vi "Measurement_UI.vi"() -> ()   [LabVIEW 2023]
uses:
  <vilib>/Instr/_visa.llb/VISA Configure Serial Port (Instr).vi
panel:
  in  "Automation Irrigation Systems":enum32{"Introverts' Garden"}(tab)
  out "Water Tension":dbl(graph)
  out "Water Tension (cbar)":dbl(knob) scale=10.0..200.0
  out "Temperature (C)":dbl(knob) scale=10.0..40.0
  out "Humidity (%)":dbl(knob) scale=0.0..100.0
  in  "Device PORT":refnum<visa-resource-name>
  in  "?":bool
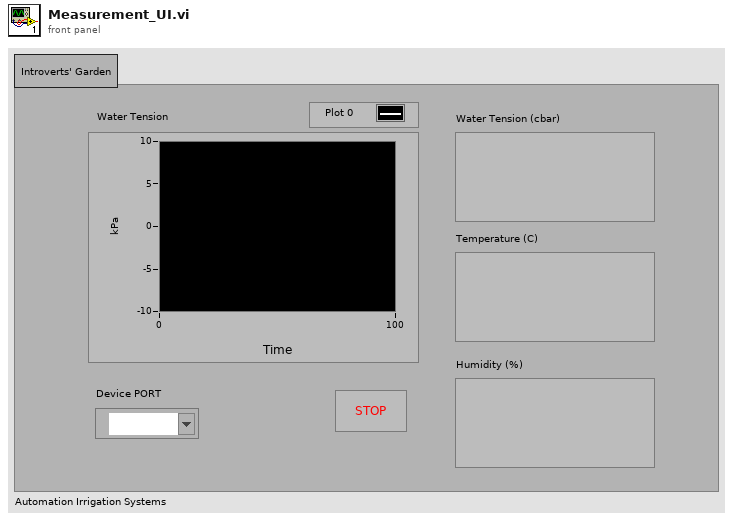
[diagram p1: front panel]
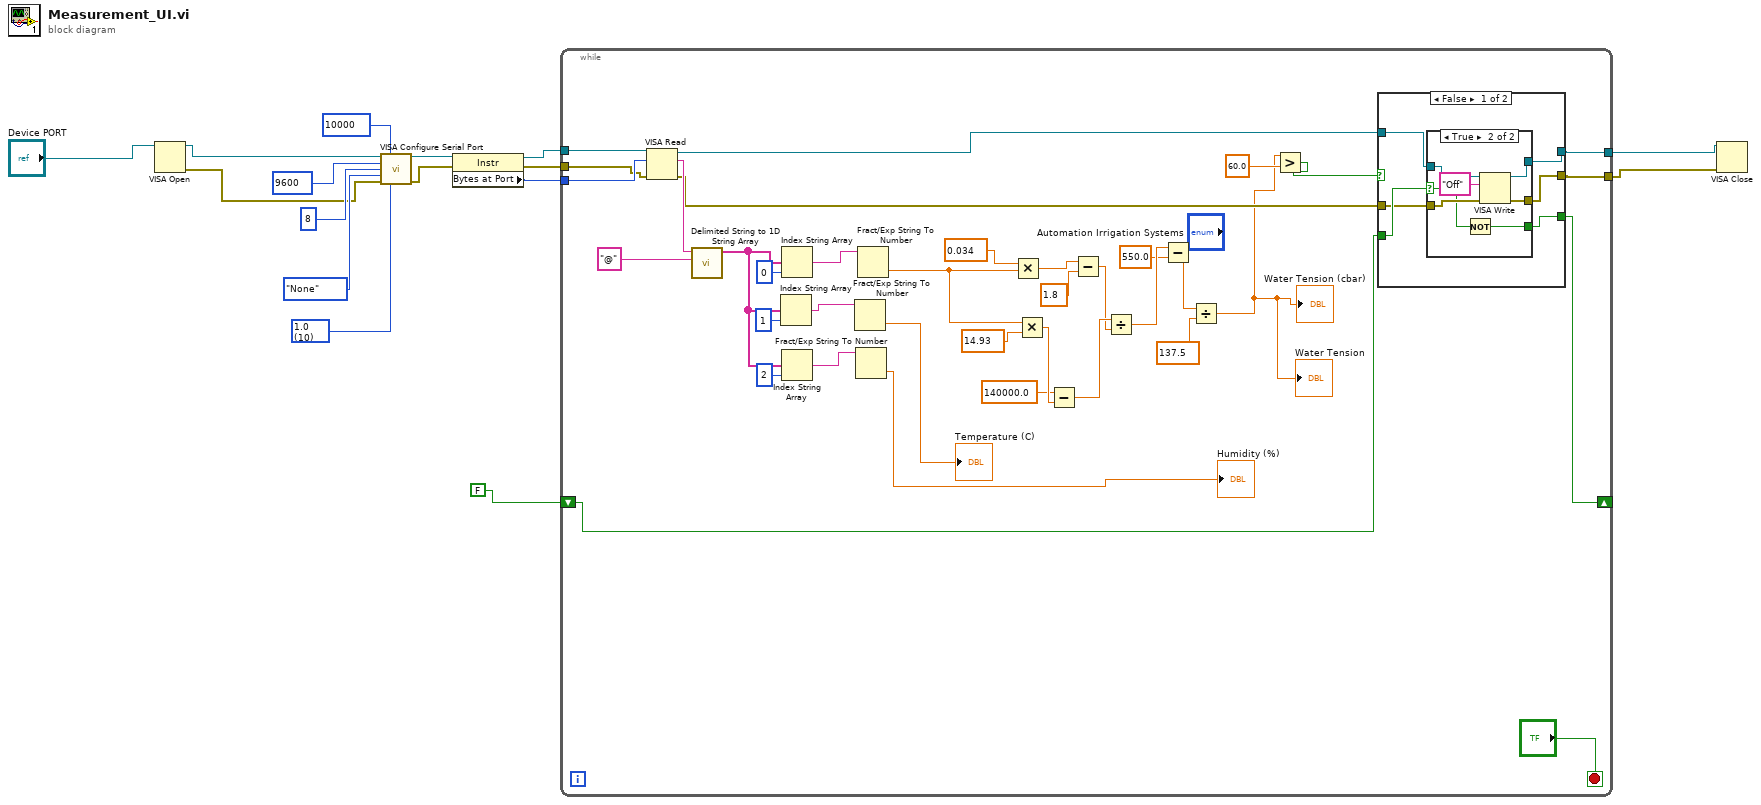
[diagram p0: block diagram]
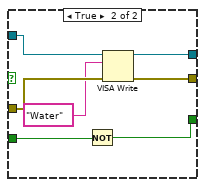
[diagram p3: hidden frame]
diagram:
  w13 = u16 10 items=["1.0"=10, "1.5"=15, "2.0"=20] ("stop bits (10: 1 bit)")
  n1 = VISA Open(VISA resource name="Device PORT") -> (VISA resource name=w10:refnum<visa-resource-name>, error out=w9:errorcluster)  [unwired: 4 in]
  n2 = call-poly "VISA Configure Serial Port"("VISA resource name"=w10, "timeout (10sec)"=u32 10000, "baud rate (9600)"=u32 9600, "data bits (8)"=u16 8, "parity (0:none)"=enum16{"None", "Odd", "Even", "Mark", "Space"}."None", "error in (no error)"=w9, "stop bits (10: 1 bit)"=w13) -> ("VISA resource name out"=w8:refnum<visa-resource-name>, "error out"=w7:errorcluster)  [unwired: 7 in]
  n3 = property class="Instr"(reference=w8, error in=w7) -> (reference out=w6:refnum<visa-resource-name>, error out=w5:errorcluster, "Bytes at Port"=w4:u32)
  n4 = while {
    tunnel: w6 -> [w53]
    tunnel: w5 -> [w51]
    tunnel: w4 -> [w52]
    tunnel: [w29] -> w3
    tunnel: [w28] -> w2
    shift-right: [w23] -> _
    shift-left: FALSE -> [w24]
    stop <- "?" stop-if-true
    n5 = VISA Read(VISA resource name=w53, byte count=w52, error in (no error)=w51) -> (VISA resource name out=w31:refnum<visa-resource-name>, read buffer=w50:string, error out=w30:errorcluster)  [unwired: 1 out]
    n6 = call <vilib>:"Delimited String to 1D String Array.vi"("delimiter"="@", "delimited string"=w50) -> ("string array"=w48:string[])  [unwired: 9 in]
    n7 = Index String Array(1:1 ("index"), 2:w48) -> (0:w43:string)  [unwired: 1 in]
    n8 = Index String Array(1:0 ("index"), 2:w48) -> (0:w44:string)  [unwired: 1 in]
    n9 = Index String Array(1:2 ("index"), 2:w48) -> (0:w42:string)  [unwired: 1 in]
    n10 = Fract/Exp String To Number(string=w43) -> (number=→"Temperature (C)":dbl)  [unwired: 3 in, 1 out]
    n11 = Fract/Exp String To Number(string=w42) -> (number=→"Humidity (%)":dbl)  [unwired: 3 in, 1 out]
    n12 = Fract/Exp String To Number(string=w44) -> (number=w40:dbl)  [unwired: 3 in, 1 out]
    n13 = Multiply(x=0.034, y=w40) -> (x*y=w22:dbl)
    n14 = Multiply(x=w40, y=14.93) -> (x*y=w38:dbl)
    n15 = Subtract(x=140000.0, y=w38) -> (x-y=w36:dbl)
    n16 = Subtract(x=w22, y=1.8) -> (x-y=w20:dbl)
    n17 = Divide(x=w36, y=w20) -> (x/y=w35:dbl)
    n18 = Subtract(x=w35, y=550.0) -> (x-y=w33:dbl)
    n19 = Divide(x=w33, y=137.5) -> (x/y=w17:dbl)
    "Water Tension (cbar)" <- w17
    "Water Tension" <- w17
    n20 = Greater?(x=w17, y=60.0) -> (0:w18:bool)
    n21 = case shown="False" w18 {
      tunnel: w31 -> [w58 w76]
      tunnel: w30 -> [w57 w75]
      tunnel: [w56 w73] -> w29
      tunnel: [w55 w72] -> w28
      tunnel: w24 -> [w59 w71]
      tunnel: [w54 w70] -> w23
      frame False {
        n22 = case shown="True" w59 {
          selector: w59 -> [w60 w65]
          tunnel: w58 -> [w62 w68]
          tunnel: w57 -> [w61 w69]
          tunnel: [w62 w67] -> w56
          tunnel: [w61 w66] -> w55
          tunnel: [w60 w64] -> w54
          frame False {
          }
          frame True {
            n23 = Not(x=w65) -> (.not. x?=w64:bool)
            n24 = VISA Write(VISA resource name=w68, write buffer="Off", error in (no error)=w69) -> (VISA resource name out=w67:refnum<visa-resource-name>, error out=w66:errorcluster)  [unwired: 1 out]
          }
        }
      }
      frame True {
        n25 = Not(x=w71) -> (.not. x?=w70:bool)
        n26 = VISA Write(VISA resource name=w76, write buffer="Water", error in (no error)=w75) -> (VISA resource name out=w73:refnum<visa-resource-name>, error out=w72:errorcluster)  [unwired: 1 out]
      }
    }
  }
  n27 = VISA Close(VISA resource name=w3, error in (no error)=w2) -> ()  [unwired: 1 out]
